vi "Set ErrorCluster.vi"(8 "error in (no error)":errorcluster, 10 "ErrorCluster":errorcluster, 11 "ErrorMessage":refnum<class "ErrorMessage.lvclass">) -> (0 "error out":errorcluster, 3 "ErrorMessage out":refnum<class "ErrorMessage.lvclass">)   [LabVIEW 2009, in "LapDog.Messaging.v2.lvlib" / "ErrorMessage.lvclass"]
doc: "Overridable accessor method for child classes to implement advanced functionality.\n\nThis method executes regardless of the error in state."
uses:
  ErrorMessage.lvclass
  ErrorMessage.lvclass/ErrorMessage.ctl
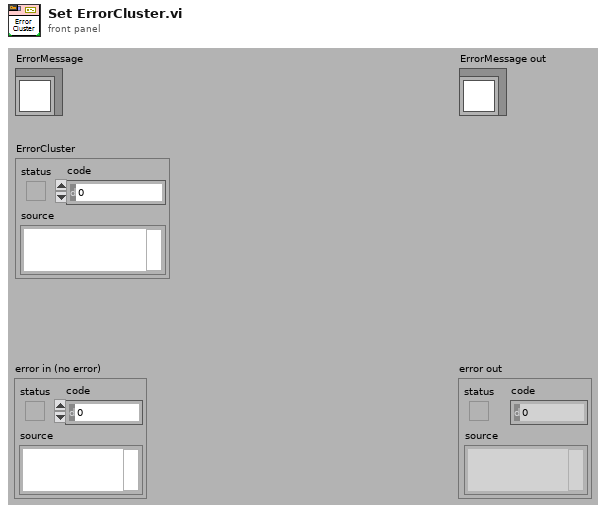
[diagram p1: front panel]
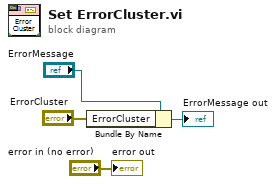
[diagram p0: block diagram]
diagram:
  n1 = Bundle By Name(cluster="ErrorMessage", "ErrorCluster"="ErrorCluster") -> (→"ErrorMessage out":refnum<class "ErrorMessage.lvclass">)
  "error out" <- "error in (no error)"
